vi "beginPrepareDoublePassPlay.vi"(9 "last command_interpreted":T1, 10 "Game":refnum<class "Game.lvclass">, 11 "PrepareDoublePassPlay in":refnum<class "PrepareDoublePassPlay.lvclass">) -> (2 "BeginPrepareDoublePass?":bool, 3 "PrepareDoublePassPlay out":refnum<class "PrepareDoublePassPlay.lvclass">)   [LabVIEW 2023, in "PrepareDoublePassPlay.lvclass"]
uses:
  PrepareDoublePassPlay.lvclass
  Game_class/Game.lvclass
  Referee_class/command_interpreted.ctl
  Game_class/Game.lvclass/Game.ctl
  Referee_class/Referee.lvclass/Referee.ctl
  Parameters_class/Parameters.lvclass/Parameters.ctl
  Game_class/Read Referee.vi
  Game_class/Read Parameters.lvclass.vi
  Game_class/Read BallRef.vi
  Game_class/Read Utilities.lvclass.vi
  Game_class/Read FieldRef.vi
  Parameters_class/Read RollToPass.vi
  Referee_class/Read command_interpreted.vi
  Referee_class/Referee.lvclass
  Parameters_class/Parameters.lvclass
  Ball_class/Ball.lvclass
  Utilities_class/Utilities.lvclass
  Field_class/Field.lvclass
panel:
  out "error out":errorcluster
  in  "error in (no error)":errorcluster
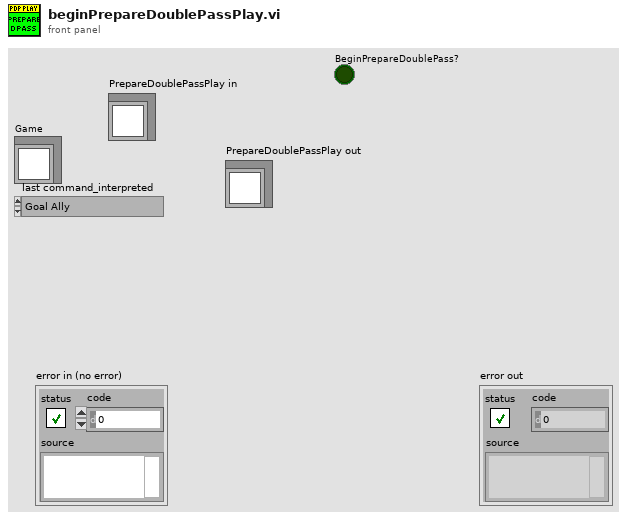
[diagram p1: front panel]
types:
  T1 = typedef "command_interpreted.ctl" = enum16{"Goal Ally", "Goal Enemy", "Ball Placement Enemy", "Ball Placement Ally", "Normal Half Time", "Extra Time  Break", "Extra Half Time", "None", "Post Game", "PKA Normal Start", "Prepare Kickoff Ally", "PKE Normal Start", "Prepare Kickoff Enemy", "Force Start", "Halt", "Timeout", "Prepare Penalty Ally", "Prepare Penalty Enemy", "PPA NormalStart", "PPE Normal Start", "Indirect Free Ally", "Direct Free Enemy", "Direct Free Ally", "Indirect Free Enemy", "Stop"}
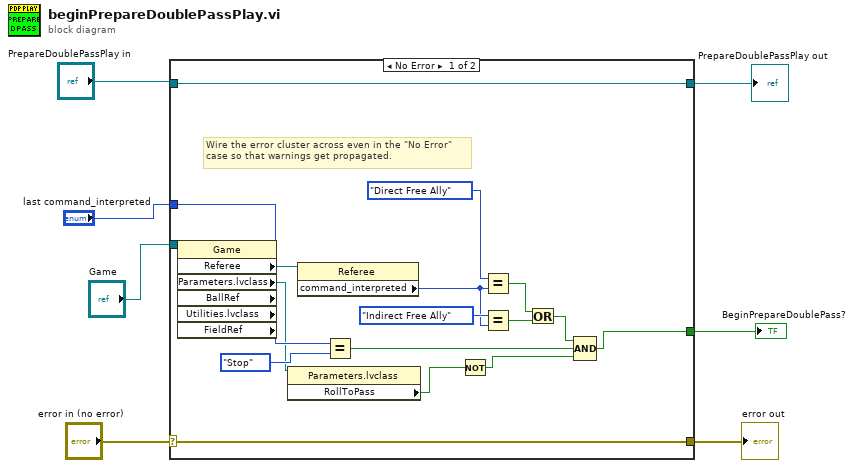
[diagram p0: block diagram]
diagram:
  n1 = case shown="No Error" "error in (no error)" {
    selector: "error in (no error)" -> [w23 w26]
    tunnel: [w23 w26] -> w6
    tunnel: [w24 w25] -> w1
    tunnel: "PrepareDoublePassPlay in" -> [w24 w25]
    tunnel: "Game" -> [w22 _]
    tunnel: [w13 _] -> w4
    tunnel: "last command_interpreted" -> [w11 _]
    frame No Error {
      # "Wire the error cluster across even in the \"No Error\"\ncase so that warnings get propagated."
      n2 = property class="Game" props=["Referee", "Parameters.lvclass", "BallRef", "Utilities.lvclass", "FieldRef"](reference=w22) -> ("Referee"=w21:refnum<class "Referee.lvclass">, "Parameters.lvclass"=w10:refnum<class "Parameters.lvclass">)  [unwired: 1 in, 5 out]
      n3 = property class="Parameters.lvclass"(reference=w10) -> ("RollToPass"=w9:bool)  [unwired: 1 in, 2 out]
      n4 = property class="Referee"(reference=w21) -> ("command_interpreted"=w17:T1)  [unwired: 1 in, 2 out]
      n5 = Equal?(x=w11, y=command_interpreted."Stop" ("command_interpreted")) -> (x = y?=w12:bool)
      n6 = Not(x=w9) -> (.not. x?=w8:bool)
      n7 = Equal?(x=command_interpreted."Direct Free Ally" ("command_interpreted"), y=w17) -> (x = y?=w16:bool)
      n8 = Equal?(x=command_interpreted."Indirect Free Ally" ("command_interpreted"), y=w17) -> (x = y?=w14:bool)
      n9 = Or(x=w16, y=w14) -> (x .or. y?=w15:bool)
      n10 = Compound Arithmetic op=AND(w15, w12, w8) -> (w13:bool)
    }
    frame Error {
    }
  }
  "error out" <- w6
  "BeginPrepareDoublePass?" <- w4
  "PrepareDoublePassPlay out" <- w1
